vi "Save Load Data(2).vi"(0 "[A/D Input]":dbl[][](array[numeric]), 11 "error in (no error)":errorcluster) -> (4 "Pass?":bool, 6 "Error Code":i32, 8 "ScaleA":i32, 10 "ScaleB":i32, 15 "error out":errorcluster)   [LabVIEW 2013]
uses:
  <vilib>/Utility/NIReport.llb/NI_report.lvclass
  <vilib>/addons/_office/excel.llb/Excel Easy Table (num).vi
  <vilib>/addons/_office/excel.llb/Excel Get Data (str).vi
  <vilib>/addons/_office/NI_ReportGenerationToolkit.lvlib
  <vilib>/Utility/NIReport.llb/Excel/NI_Excel.lvclass
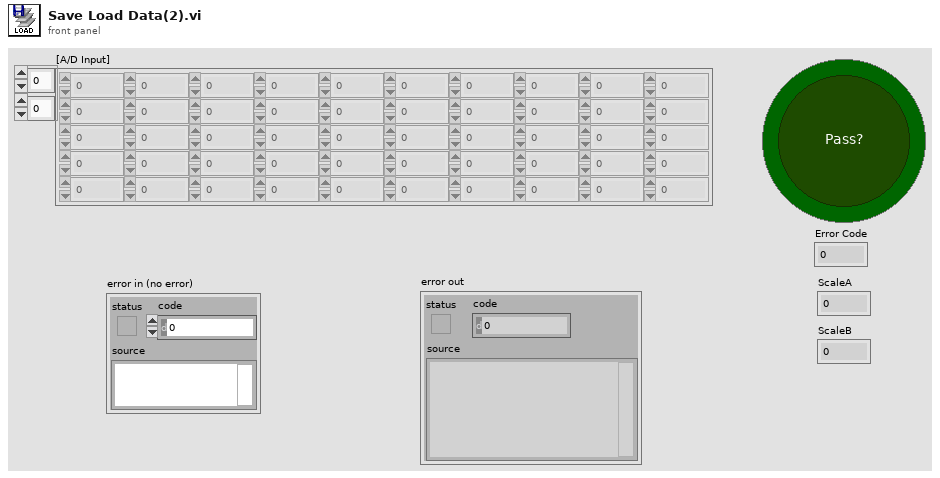
[diagram p1: front panel]
types:
  T1 = enum16{"maximized", "minimized", "normal", "no change"}
  T2 = enum16{"Standard Report", "HTML", "Word", "Excel"}
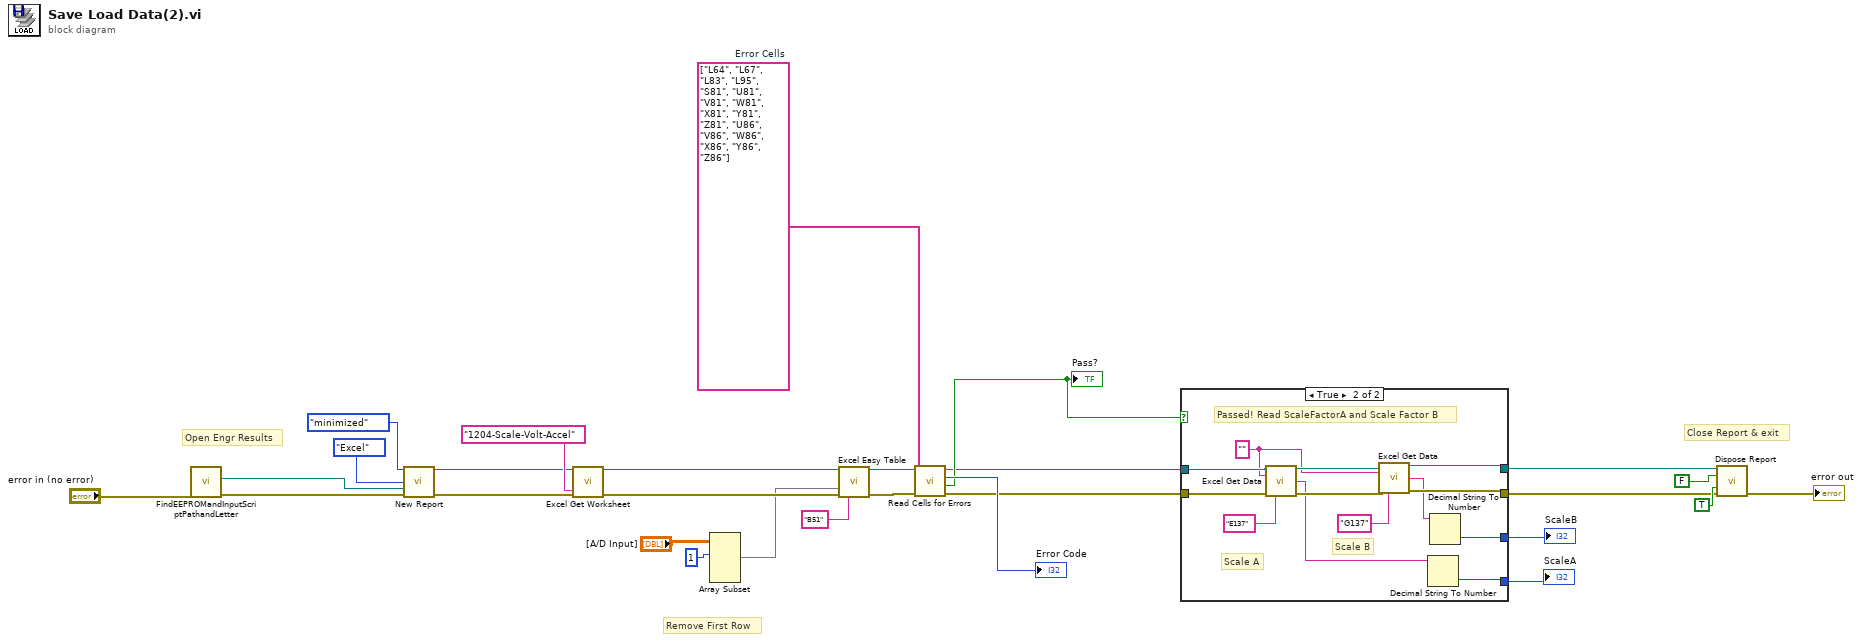
[diagram p0: block diagram]
diagram:
  w10 = string[] ["L64", "L67", "L83", "L95", "S81", "U81", "V81", "W81", "X81", "Y81", "Z81", "U86", "V86", "W86", "X86", "Y86", "Z86"]  # Error Cells
  # "Remove First Row"
  # "Close Report & exit"
  # "Open Engr Results"
  n1 = call "FindEEPROMandInputScriptPathandLetter.vi"("Error In"="error in (no error)") -> ("Error Out"=w18:errorcluster, "Engr Result Path"=w28:path)  [unwired: 6 in, 1 out]
  n2 = call <vilib>:"New Report.vi"("window state (normal)"=T1."minimized", "report type"=T2."Excel", "template (empty)"=w28, "error in (no error)"=w18) -> ("report out"=w21:refnum<class "NI_report.lvclass">, "error out"=w20:errorcluster)  [unwired: 10 in]
  n3 = call <vilib>:"Excel Get Worksheet.vi"("report in"=w21, "error in (no error)"=w20, "name (\"\")"="1204-Scale-Volt-Accel" ("name (\"\")")) -> ("report out"=w17:refnum<class "NI_report.lvclass">, "error out"=w16:errorcluster)  [unwired: 11 in]
  n4 = Array Subset(array="[A/D Input]", index (row)=1 ("length")) -> (w9:dbl[][])  [unwired: 3 in]
  n5 = call-poly <vilib>:"Excel Easy Table.vi"("report in"=w17, "text data"=w9, "error in (no error)"=w16, "name (\"\")"="B51" ("name (\"\")")) -> ("report out"=w14:refnum<class "NI_report.lvclass">, "error out"=w15:errorcluster)  [unwired: 7 in, 3 out]
  n6 = call "Read Cells for Errors.vi"("error in (no error)"=w15, "Error Cells (ex:A12)"=w10, "NI_report in"=w14) -> ("error out"=w7:errorcluster, "Pass?"=w8:bool, "Error Code"=→"Error Code":i32, "NI_report out"=w6:refnum<class "NI_report.lvclass">)  [unwired: 5 in]
  "Pass?" <- w8
  n7 = case shown="True" w8 {
    tunnel: w7 -> [w29 w43]
    tunnel: w6 -> [w30 w42]
    tunnel: [w30 w39] -> w5
    tunnel: [w29 w38] -> w4
    tunnel: [_ w31] -> w3
    tunnel: [_ w32] -> w2
    frame False {
      # "Fail. No need to read the Scale Values"
    }
    frame True {
      w36 = "" ("name (\"\")")
      # "Scale A"
      # "Scale B"
      # "Passed! Read ScaleFactorA and Scale Factor B"
      n8 = call-poly <vilib>:"Excel Get Data.vi"("report in"=w42, "data type"=w36, "error in (no error)"=w43, "name (\"\")"="E137" ("name (\"\")")) -> ("report out"=w40:refnum<class "NI_report.lvclass">, "data"=w34:string, "error out"=w41:errorcluster)  [unwired: 9 in]
      n9 = call-poly <vilib>:"Excel Get Data.vi"("report in"=w40, "data type"=w36, "error in (no error)"=w41, "name (\"\")"="G137" ("name (\"\")")) -> ("report out"=w39:refnum<class "NI_report.lvclass">, "data"=w35:string, "error out"=w38:errorcluster)  [unwired: 9 in]
      n10 = Decimal String To Number(string=w34) -> (number=w31:i32)  [unwired: 2 in, 1 out]
      n11 = Decimal String To Number(string=w35) -> (number=w32:i32)  [unwired: 2 in, 1 out]
    }
  }
  "ScaleA" <- w3
  "ScaleB" <- w2
  n12 = call-dynamic "Dispose Report.vi"("report in"=w5, "wait until printing completed? (T)"=FALSE, "save changes? (F)"=TRUE, "error in (no error)"=w4) -> ("error out"=→"error out":errorcluster)  [unwired: 11 in]
